vi "Actor Core.vi"(8 "error in":errorcluster, 11 "QuickNote in":refnum<class "QuickNote.lvclass">) -> (0 "error out":errorcluster, 3 "Actor out":refnum<class "Actor.lvclass">)   [LabVIEW 2020]
doc: "(<B>Filename</B>: Actor Framework.lvlib:Actor.lvclass:Actor Core.vi)\n\nReceives messages to the actor, reacts to them, and initiates any error handling that may shut the actor down.\n\nDescendant classes may override this VI to append parallel tasks for the actor to complete while it handles messages. Overrides use the Call Parent Class Method node."
uses:
  <vilib>/ActorFramework/Actor/Actor.lvclass
  QuickNoteUI/QuickNoteUI.lvclass
  QuickNote.lvclass
  E:/Development/DevHardSoftware/MicroscopyFramework/Analyser/Analyser/Analyser.lvclass
  C:/Program Files/National Instruments/LabVIEW 2020/vi.lib/ActorFramework/Actor/Actor.lvclass
  E:/Development/DevHardSoftware/MicroscopyFramework/QuickNote/QuickNote/QuickNote.lvclass
  E:/Development/DevHardSoftware/MicroscopyFramework/QuickNoteUI/QuickNoteUI.lvclass
  E:/Development/DevHardSoftware/MicroscopyFramework/Interface/DataListener/DataListener.lvclass
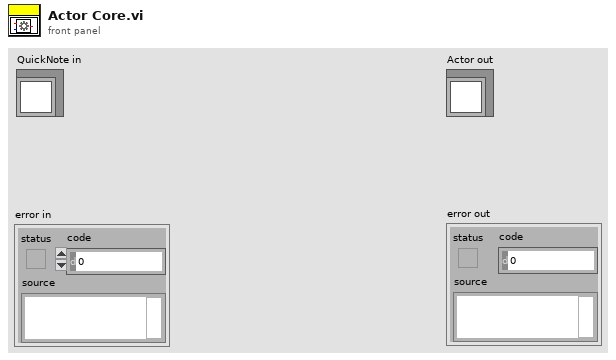
[diagram p1: front panel]
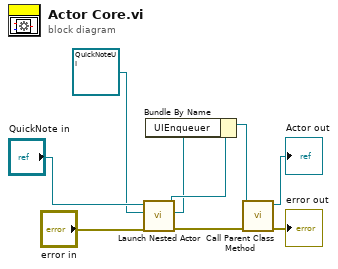
[diagram p0: block diagram]
diagram:
  n1 = call <vilib>:"Launch Nested Actor.vi"("error in (no error)"="error in", "Nested Actor"=refnum<class "QuickNoteUI.lvclass"> refnum ("QuickNote.lvlib:QuickNoteUI.lvlib:QuickNoteUI.lvclass"), "Caller Actor in"="QuickNote in") -> ("error out"=w6:errorcluster, "Nested Actor's Enqueuer"=w1:refnum<class "Message Enqueuer.lvclass">, "Caller Actor out"=w4:refnum<class "QuickNote.lvclass">)  [unwired: 6 in]
  n2 = Bundle By Name(cluster=w4, "UIEnqueuer"=w1) -> (w2:refnum<class "QuickNote.lvclass">)
  n3 = call-parent "Call Parent Class Method"("error in"=w6, "Actor in"=w2) -> ("error out"=→"error out":errorcluster, "Actor out"=→"Actor out":refnum<class "Actor.lvclass">)  [unwired: 8 in]
